vi "Write State.vi"(8 "error in (no error)":errorcluster, 10 "State":T1, 11 "BiStableShutter in":refnum<class "BiStableShutter.lvclass">) -> (0 "error out":errorcluster, 3 "BiStableShutter out":refnum<class "BiStableShutter.lvclass">)   [LabVIEW 2016, in "BiStableShutter.lvclass"]
uses:
  BiStableShutter.lvclass
  Controls/Shutter States.ctl
  Shutter.lvclass
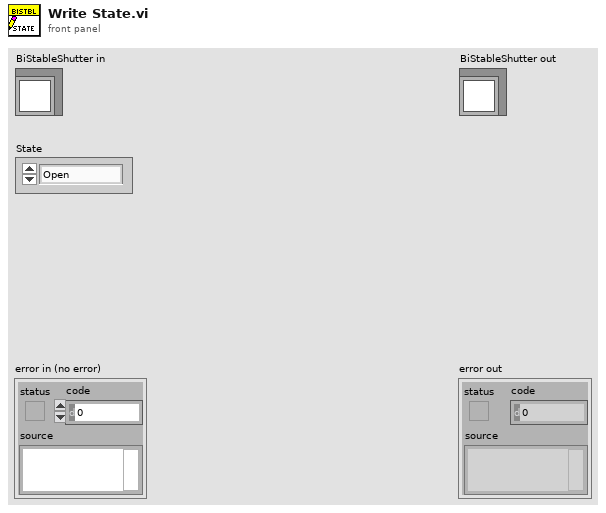
[diagram p1: front panel]
types:
  T1 = typedef "Shutter States.ctl" = enum16{"Open", "Close", "Wait", "Off", "Arm", "Idle"}
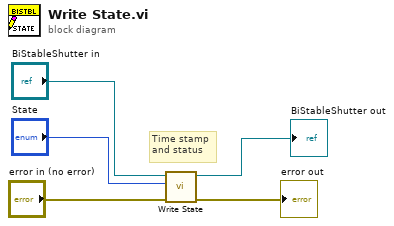
[diagram p0: block diagram]
diagram:
  # "Time stamp\nand status"
  n1 = call-parent "Write State.vi"("error in (no error)"="error in (no error)", "Set"="State", "Shutter in"="BiStableShutter in") -> ("error out"=→"error out":errorcluster, "Shutter out"=→"BiStableShutter out":refnum<class "BiStableShutter.lvclass">)  [unwired: 7 in]
